vi "m1m3_registerCallback_logEvent_PIDInfo.vi"(8 "error in (no error)":errorcluster, 10 "skipOld":bool, 11 "handle":i32) -> (0 "error out":errorcluster, 3 "function return":i32)   [LabVIEW 2016, in "SALLV_m1m3.lvlib"]
doc: "int m1m3_shm_registerCallback_logevent_PIDInfoLV(int handle, bool skipOld);"
uses:
  SALLV_m1m3.lvlib
  SALLV_m1m3.so
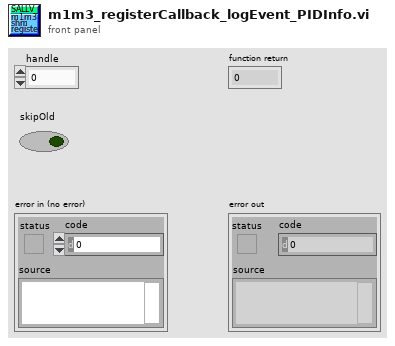
[diagram p1: front panel]
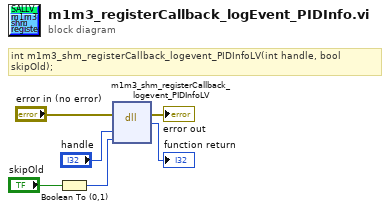
[diagram p0: block diagram]
diagram:
  # "int m1m3_shm_registerCallback_logevent_PIDInfoLV(int handle, bool skipOld);"
  n1 = Boolean To (0,1)(Boolean="skipOld") -> (0, 1=w3:i16)
  n2 = dll-call lib="opt/CODE/SALLV_m1m3/SALLV_m1m3.*" fn="m1m3_shm_registerCallback_logevent_PIDInfoLV"(error in="error in (no error)", "handle"="handle", "skipOld"=w3) -> (error out=→"error out":errorcluster, →"function return":i32)  [unwired: 4 in, 1 out]
